vi "NI-DAQmxBaseKernel.vi"() -> (0 "Error Out":errorcluster)   [LabVIEW 2020]
uses:
  Globals/Meas_global.vi
  PWA/PWAtasksGLOBAL.vi
  <vilib>/_DAQmxBase/Internals/DAQmxBase Create Channel (AI-Voltage-Basic).vi
  <vilib>/_DAQmxBase/Internals/DAQmxBase Timing (Sample Clock).vi
  <vilib>/_DAQmxBase/Internals/DAQmxBase Read (Analog 2D DBL NChan NSamp).vi
  Sub_vis/Upload Data.ctl
panel:
  in  "Half-span(V)":dbl=10.0 format="%#_13g"
  out "FsRead":dbl
  out "FsReq":dbl
  out "CurrentBlock":i32
  out "Case":string
  out "Audit Trail":string[](array[string])
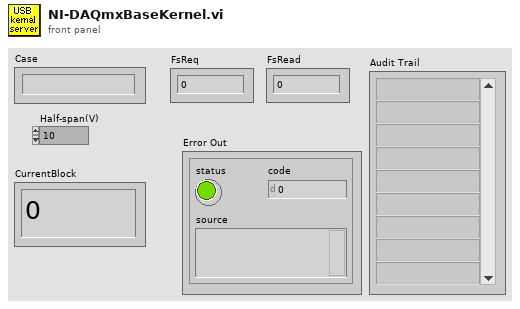
[diagram p1: front panel]
types:
  T1 = typedef "Analysis_info_cluster.ctl" = cluster{"Colour":u32, "Inst type":T2, "Inst name":string, "Symbol":string, "Code name":string, "Extra Info":string, "Inst Array":T3, "Extra Titles":string[], "Extra Values":string[], "U":dbl, "u^2":dbl, "u^3":dbl, "u^4":dbl, "Skew_u":dbl, "Kurt_u":dbl, "Sd Error in Mean":dbl, "% u'/U":dbl, "X":dbl, "Y":dbl, "Z":dbl, "Timescale integral Estimate":dbl, "Sd Error in Variance":dbl, "Calib File":path, "Calib Constants":dbl[], "Output Position":bool, "Stats":enum16{"None", "Basic", "Full"}, "Av Sampling Rate":dbl, "Av No of Samples":dbl, "Total Meas Time (s)":dbl, "ADAM Ch Name":string, "Max value":dbl, "Min value":dbl, "Req Sample Rate Hz":dbl, "Sync Delay Time (s)":dbl, "Ch No":i16, "Device":string, "Use Latest Calib":bool, "Port":string, "Metadata Ch Names":string[], "Metadata Ch Values":string[], "Label":string}
  T2 = typedef "Inst_type.ctl" = enum16{"Raw voltage", "Raw with zero offsetting", "Propeller anemometer", "Pressure Transducer", "Pitot-static tube", "Hot wire", "Cross wire 1", "Cross wire 2", "Generic Linear", "Generic Polynomial", "Generic BackPoly", "Fast FID", "Thermocouple", "Cold wire", "Pulsed Wire", "LDA Vel", "LDA Tran time", "LDA Arr time", "Microphone"}
  T3 = typedef "Instrument_Array.ctl" = enum16{"PWA", "LDA", "Analogue"}
  T4 = typedef "Device ID port info.ctl" = cluster{"Ch No":i16[], "Req Sampling Rate":dbl[], "Port":string, "Index":i32[]}
  T5 = typedef "Upload Data.ctl" = enum16{"Voltage Array", "Time Trace Cluster"}
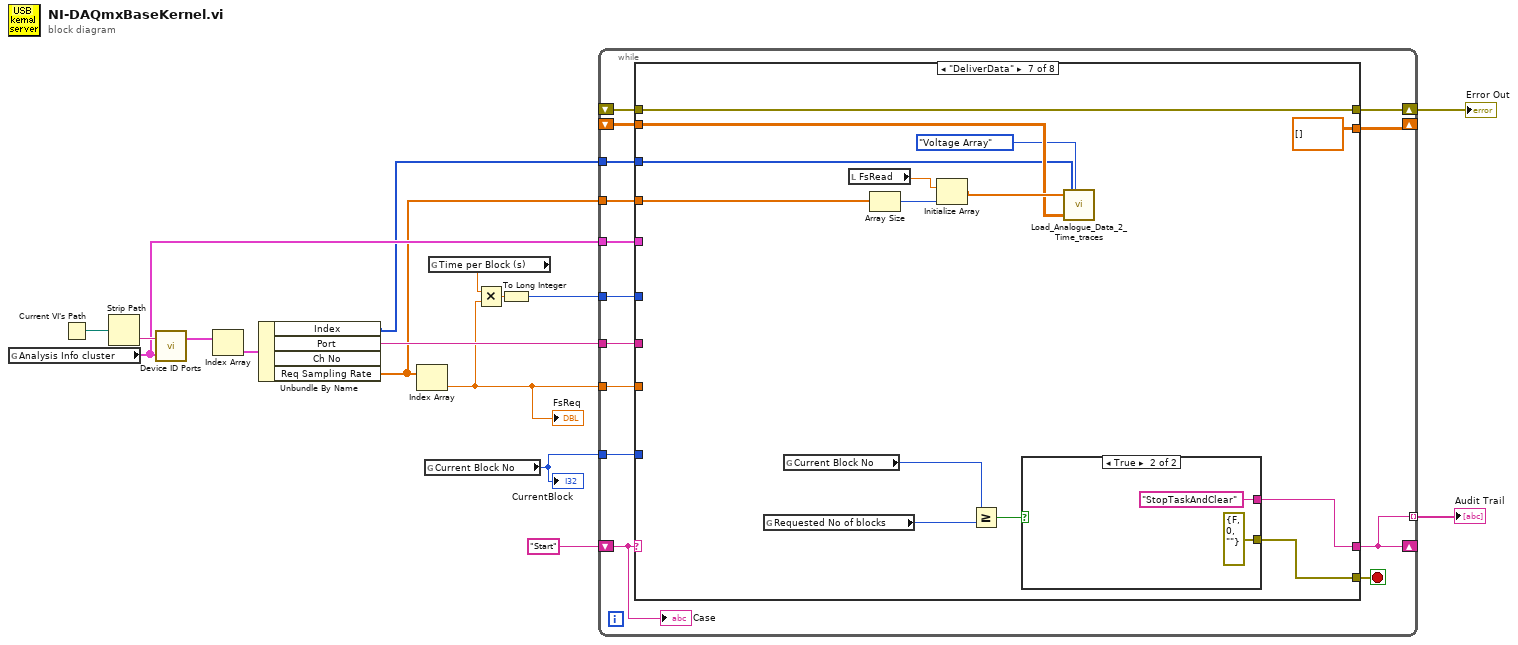
[diagram p0: block diagram]
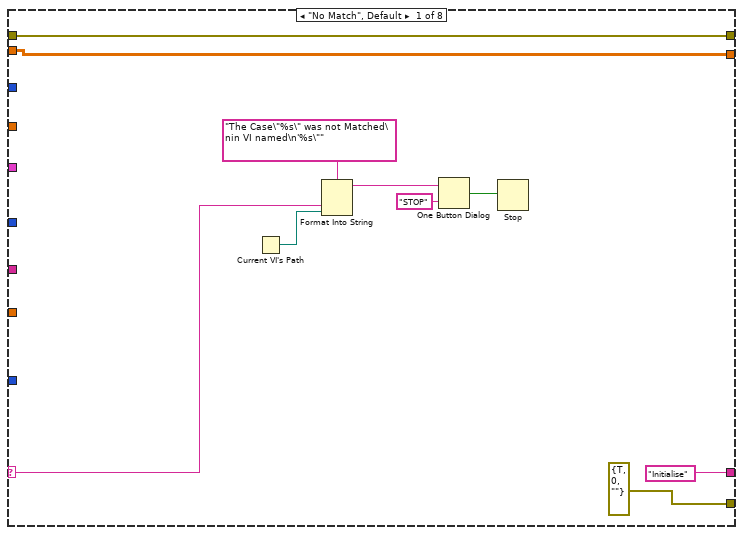
[diagram p2: hidden frame]
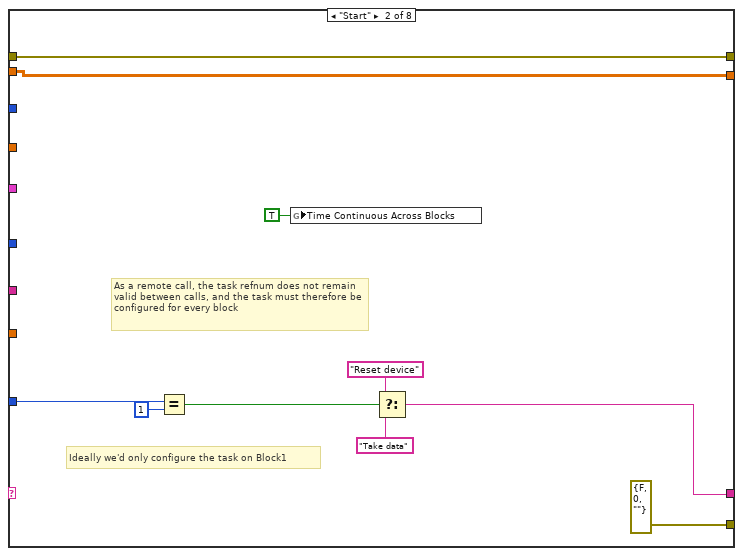
[diagram p3: hidden frame]
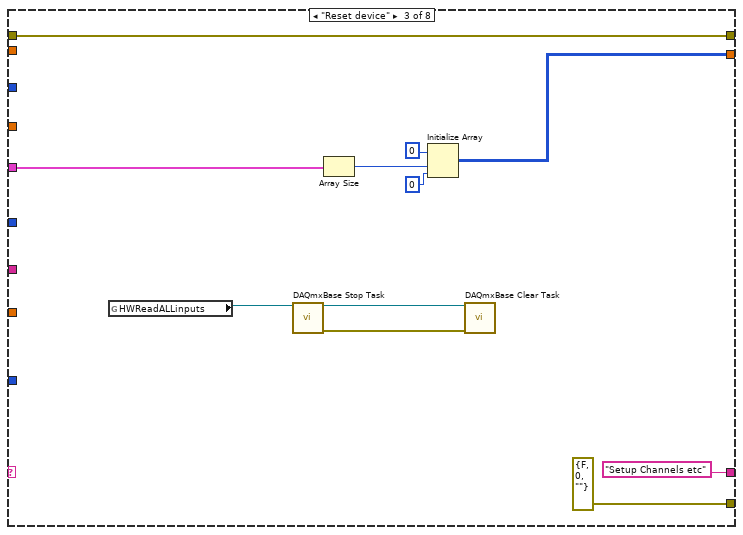
[diagram p4: hidden frame]
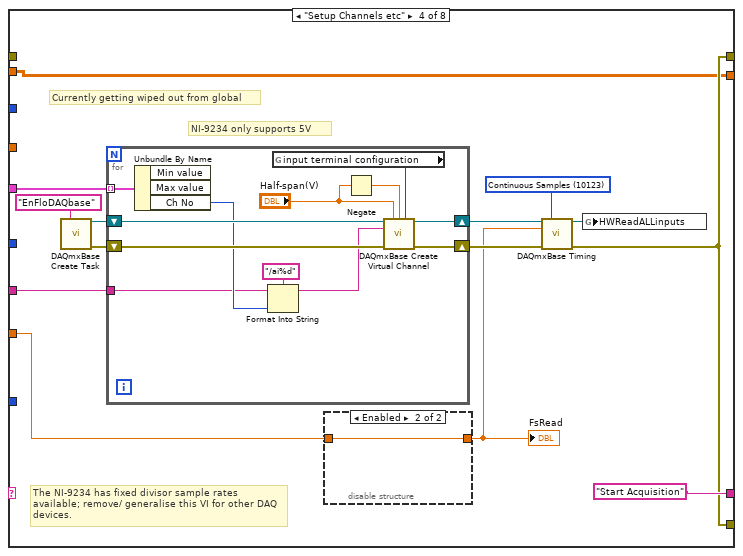
[diagram p5: hidden frame]
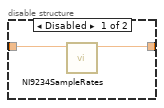
[diagram p6: hidden frame]
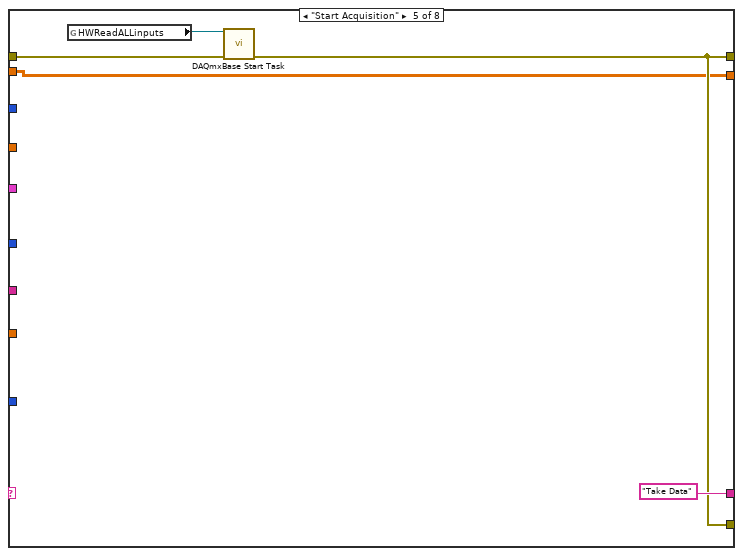
[diagram p7: hidden frame]
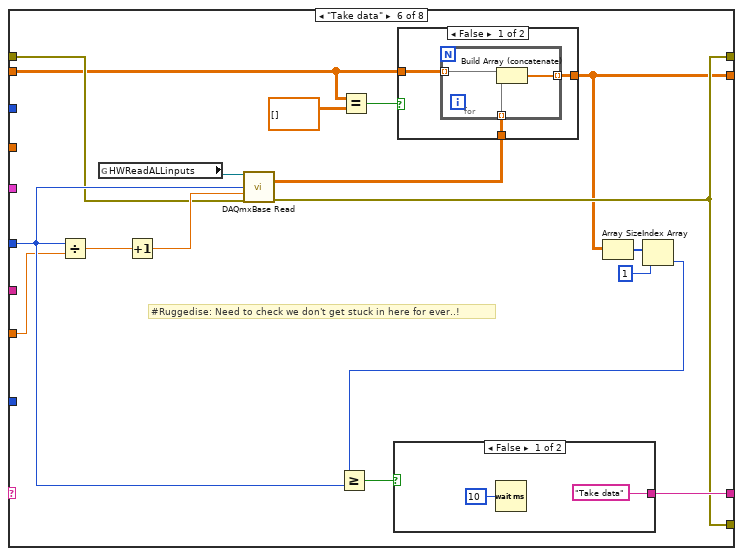
[diagram p8: hidden frame]
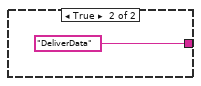
[diagram p10: hidden frame]
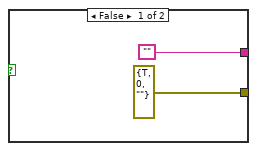
[diagram p11: hidden frame]
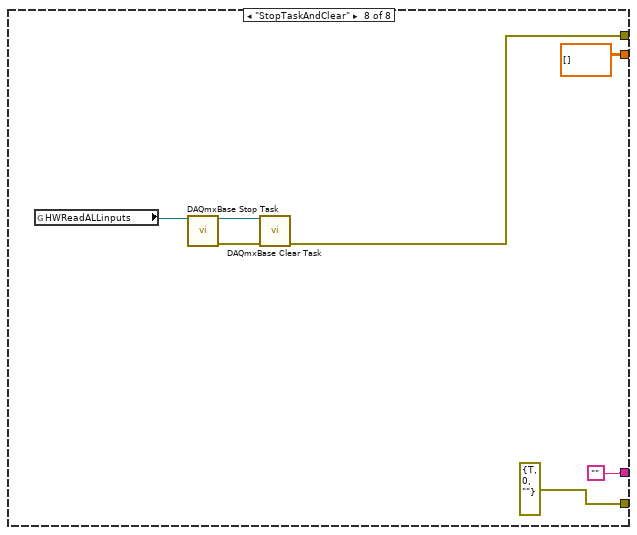
[diagram p12: hidden frame]
diagram:
  n1 = global read "Meas_global.vi" "Analysis Info cluster"() -> (w6:T1[])
  n2 = Current VI's Path() -> (path=w9:path)
  n3 = Strip Path(path=w9) -> (name=w10:string)  [unwired: 1 out]
  n4 = call "Device ID Ports.vi"("Analysis Info cluster"=w6, "Device ID"=w10) -> ("Device port info"=w11:T4[])  [unwired: 1 out]
  n5 = Index Array(array=w11) -> (element=w12:T4)  [unwired: 1 in]
  n6 = Unbundle By Name(w12) -> ("Index"=w2:i32[], "Port"=w5:string, "Req Sampling Rate"=w1:dbl[])  [unwired: 1 out]
  n7 = Index Array(array=w1) -> (element=w3:dbl)  [unwired: 1 in]
  "FsReq" <- w3
  n8 = global read "Meas_global.vi" "Current Block No"() -> (w13:i32)
  "CurrentBlock" <- w13
  n9 = global read "Meas_global.vi" "Time per Block (s)"() -> (w7:dbl)
  n10 = Multiply(x=w7, y=w3) -> (x*y=w8:dbl)
  n11 = To Long Integer(number=w8) -> (32bit integer=w4:i32)
  n12 = while {
    shift-left: "Start" -> [w21]
    shift-right: [w22] -> _
    shift-right: [w29] -> w15
    shift-left: _ -> [w28]
    tunnel: w4 -> [w27]
    tunnel: w13 -> [w26]
    tunnel: w6 -> [w25]
    shift-right: [w23] -> _
    shift-left: _ -> [w24]
    tunnel: [w22] -> w14 mode=indexing
    tunnel: w3 -> [w20]
    tunnel: w5 -> [w19]
    tunnel: w2 -> [w18]
    tunnel: w1 -> [w17]
    stop <- w30 stop-if-true
    n13 = case shown="\"DeliverData\"" w21 {
      selector: w21 -> [w32 _ _ _ _ _ _ _]
      tunnel: [errorcluster {"status"=TRUE, "code"=0, "source"=""} ("error out") errorcluster {"status"=FALSE, "code"=0, "source"=""} ("error out") errorcluster {"status"=FALSE, "code"=0, "source"=""} ("error out") w68 w93 w107 w134 errorcluster {"status"=TRUE, "code"=0, "source"=""} ("error out")] -> w30
      tunnel: ["Initialise" w48 "Setup Channels etc" "Start Acquisition" "Take Data" w111 w135 ""] -> w22
      tunnel: [w33 w50 w59 w68 w93 w107 w136 w142] -> w29
      tunnel: w28 -> [w33 w50 w59 _ w94 w101 w136 _]
      tunnel: w27 -> [_ _ _ _ _ w109 _ _]
      tunnel: w26 -> [_ w43 _ _ _ _ _ _]
      tunnel: w25 -> [_ _ w52 w70 _ _ _ _]
      tunnel: w24 -> [w31 w45 _ w67 w92 w98 w126 _]
      tunnel: [w31 w45 w51 w67 w92 w102 dbl[][] [] dbl[][] []] -> w23
      tunnel: w20 -> [_ _ _ w63 _ w96 _ _]
      tunnel: w19 -> [_ _ _ w64 _ _ _ _]
      tunnel: w18 -> [_ _ _ _ _ _ w125 _]
      tunnel: w17 -> [_ _ _ _ _ _ w124 _]
      frame "No Match", Default {
        n14 = Current VI's Path() -> (path=w35:path)
        n15 = Format Into String(format string="The Case\"%s\" was not Matched\nin VI named\n'%s\"" ("Format String"), w32, w35) -> (resulting string=w38:string)  [unwired: 2 in, 1 out]
        n16 = One Button Dialog(message=w38, button name ("OK")="STOP") -> (true=w36:bool)
        n17 = Stop(stop? (T)=w36) -> ()
      }
      frame "Start" {
        # "Ideally we'd only configure the task on Block1"
        # "As a remote call, the task refnum does not remain valid between calls, and the task must therefore be configured for every block"
        n18 = Equal?(x=w43, y=1) -> (x = y?=w41:bool)
        n19 = global write "Meas_global.vi" "Time Continuous Across Blocks"(TRUE ("Time Continuous Across Blocks")) -> ()
        n20 = Select(t="Reset device", s=w41, f="Take data") -> (s? t:f=w48:string)
      }
      frame "Reset device" {
        n21 = global read "PWAtasksGLOBAL.vi" "HWReadALLinputs"() -> (w57:refnum<k21>)
        n22 = call <vilib>:"DAQmxBase Stop Task.vi"("task/channels in"=w57) -> ("task out"=w61:refnum<k21>, "error out"=w60:errorcluster)  [unwired: 13 in]
        n23 = Array Size(array=w52) -> (size(s)=w54:i32)
        n24 = Initialize Array(i16 0, w54, 0 ("dimension size")) -> (w51:i16[][])
        n25 = call <vilib>:"DAQmxBase Clear Task.vi"("task in"=w61, "error in"=w60) -> ()  [unwired: 13 in, 1 out]
      }
      frame "Setup Channels etc" {
        w73 = 10123 items=["Finite Samples"=10178, "Continuous Samples"=10123, "Hardware Timed Single Point"=12522] ("sample mode")
        # "NI-9234 only supports 5V"
        # "Currently getting wiped out from global"
        # "The NI-9234 has fixed divisor sample rates available; remove/ generalise this VI for other DAQ devices."
        n26 = call <vilib>:"DAQmxBase Create Task.vi"("new task name"="EnFloDAQbase") -> ("task out"=w71:refnum<k21>, "error out"=w74:errorcluster)  [unwired: 13 in]
        n27 = for {
          tunnel: w70 -> [w90] mode=indexing
          shift-right: [w88] -> w72
          shift-left: w71 -> [w89]
          shift-right: [w87] -> w75
          shift-left: w74 -> [w86]
          tunnel: w64 -> [w81]
          n28 = Unbundle By Name(w90) -> ("Ch No"=w83:i16)  [unwired: 2 out]
          n29 = Format Into String(format string="/ai%d", initial string=w81, w83) -> (resulting string=w82:string)  [unwired: 1 in, 1 out]
          n30 = global read "Meas_global.vi" "input terminal configuration"() -> (w85:i32)
          n31 = Negate(x="Half-span(V)") -> (-x=w80:dbl)
          n32 = call-poly <vilib>:"DAQmxBase Create Virtual Channel.vi"("task in"=w89, "maximum value"="Half-span(V)", "minimum value"=w80, "input terminal configuration"=w85, "physical channels"=w82, "error in"=w86) -> ("task out"=w88:refnum<k21>, "error out"=w87:errorcluster)  [unwired: 8 in]
        }
        n33 = disable-structure shown="Enabled" {
          disable-tunnel: w63 -> [w77 w78]
          disable-tunnel: [w76 w78] -> w62
          frame Disabled {
            n34 = call "NI9234SampleRates.vi"("RequestedFrequency(Hz)"=w77) -> ("ClosestHigherFrequency(Hz)"=w76:dbl)  [unwired: 10 in]
          }
          frame Enabled {
          }
        }
        "FsRead" <- w62
        n35 = call-poly <vilib>:"DAQmxBase Timing.vi"("task/channels in"=w72, "sample mode"=w73, "rate"=w62, "error in"=w75) -> ("task out"=w65:refnum<k21>, "error out"=w68:errorcluster)  [unwired: 10 in]
        n36 = global write "PWAtasksGLOBAL.vi" "HWReadALLinputs"(w65) -> ()
      }
      frame "Start Acquisition" {
        n37 = global read "PWAtasksGLOBAL.vi" "HWReadALLinputs"() -> (w91:refnum<k21>)
        n38 = call <vilib>:"DAQmxBase Start Task.vi"("task/channels in"=w91, "error in"=w94) -> ("error out"=w93:errorcluster)  [unwired: 12 in, 1 out]
      }
      frame "Take data" {
        # "#Ruggedise: Need to check we don't get stuck in here for ever..!"
        n39 = Divide(x=w109, y=w96) -> (x/y=w112:dbl)
        n40 = global read "PWAtasksGLOBAL.vi" "HWReadALLinputs"() -> (w100:refnum<k21>)
        n41 = Increment(x=w112) -> (x+1=w108:dbl)
        n42 = call-poly <vilib>:"DAQmxBase Read.vi"("task/channels in"=w100, "number of samples per channel"=w109, "timeout"=w108, "error in"=w101) -> ("data"=w103:dbl[][], "error out"=w107:errorcluster)  [unwired: 9 in, 1 out]
        n43 = Equal?(x=w98, y=dbl[][] []) -> (x = y?=w97:bool)
        n44 = case shown="False" w97 {
          tunnel: w103 -> [w115 w119]
          tunnel: w98 -> [w114 _]
          tunnel: [w113 w119] -> w102
          frame False {
            n45 = for {
              tunnel: w115 -> [w118] mode=indexing
              tunnel: w114 -> [w117] mode=indexing
              tunnel: [w116] -> w113 mode=indexing
              n46 = Build Array (concatenate)(w117, w118) -> (w116:dbl[])
            }
          }
          frame True {
          }
        }
        n47 = Array Size(array=w102) -> (size(s)=w105:i32[])
        n48 = Index Array(array=w105, index=1) -> (element=w104:i32)
        n49 = Greater Or Equal?(x=w104, y=w109) -> (x >= y?=w110:bool)
        n50 = case shown="False" w110 {
          tunnel: ["Take data" "DeliverData"] -> w111
          frame False {
            n51 = Wait (ms)(milliseconds to wait=u32 10) -> ()  [unwired: 1 out]
          }
          frame True {
          }
        }
      }
      frame "DeliverData" {
        n52 = global read "Meas_global.vi" "Requested No of blocks"() -> (w133:i32)
        n53 = global read "Meas_global.vi" "Current Block No"() -> (w132:i32)
        n54 = local read "FsRead"() -> (w127:dbl)
        n55 = Array Size(array=w124) -> (size(s)=w129:i32)
        n56 = Initialize Array(w127, w129) -> (w128:dbl[])
        n57 = Greater Or Equal?(x=w132, y=w133) -> (x >= y?=w131:bool)
        n58 = case shown="True" w131 {
          tunnel: ["" "StopTaskAndClear"] -> w135
          tunnel: [errorcluster {"status"=TRUE, "code"=0, "source"=""} ("error out") errorcluster {"status"=FALSE, "code"=0, "source"=""} ("error out")] -> w134
          frame False {
          }
          frame True {
          }
        }
        n59 = call "Load_Analogue_Data_2_Time_traces.vi"("Sampling Rate (Hz)"=w128, "Mode"=Upload_Data."Voltage Array", "Index"=w125, "Voltage Array"=w126) -> ()  [unwired: 3 in]
      }
      frame "StopTaskAndClear" {
        n60 = global read "PWAtasksGLOBAL.vi" "HWReadALLinputs"() -> (w145:refnum<k21>)
        n61 = call <vilib>:"DAQmxBase Stop Task.vi"("task/channels in"=w145) -> ("task out"=w147:refnum<k21>, "error out"=w146:errorcluster)  [unwired: 13 in]
        n62 = call <vilib>:"DAQmxBase Clear Task.vi"("task in"=w147, "error in"=w146) -> ("error out"=w142:errorcluster)  [unwired: 13 in]
      }
    }
    "Case" <- w21
  }
  "Error Out" <- w15
  "Audit Trail" <- w14
